vi "camToPipette_abs_3d.vi"(7 "which manipulator":T2(ring), 9 "transform cluster + actuator":T1, 10 "current positions":T3, 11 "abs pixel location":dbl[](array[numeric])) -> (3 "pipette location (steps)":dbl[](array[numeric]))   [LabVIEW 2015]
uses:
  pipette cleaning/pressure box/cleaning_soft/controls/actuator_type.ctl
  pipette cleaning/pressure box/cleaning_soft/controls/actuator_cluster.ctl
  transform_properties_actuators.ctl
  controls/transform_cluster_actuator.ctl
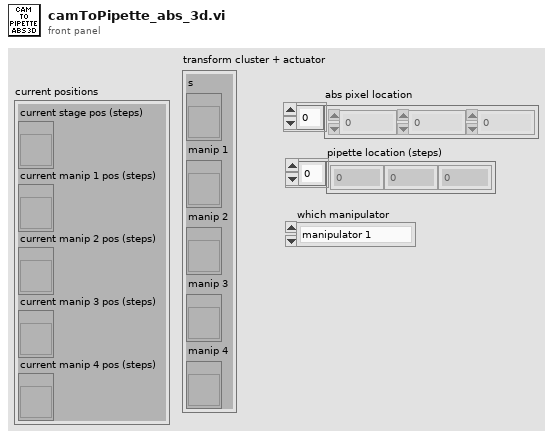
[diagram p1: front panel]
types:
  T1 = typedef "transform_cluster_actuator.ctl" = cluster{"s":refnum<vi>, "manip 1":refnum<vi>, "manip 2":refnum<vi>, "manip 3":refnum<vi>, "manip 4":refnum<vi>}
  T2 = enum16{"manipulator 1", "manipulator 2", "manipulator 3", "manipulator 4"}
  T3 = cluster{"current stage pos (steps)":refnum<vi>, "current manip 1 pos (steps)":refnum<vi>, "current manip 2 pos (steps)":refnum<vi>, "current manip 3 pos (steps)":refnum<vi>, "current manip 4 pos (steps)":refnum<vi>}
  T4 = typedef "transform_properties_actuators.ctl" = cluster{"theta (deg)":dbl, "X sc factor (px/step)":dbl, "Y sc factor (px/step)":dbl, "zero loc (x,y,z)":dbl[], "flip y?":bool, "flip x?":bool, "gamma (deg)":dbl, "flip z?":bool, "Z sc factor (px/step)":dbl, "actuator":T5, "safe space (steps)":i32[]}
  T5 = typedef "actuator_cluster.ctl" = cluster{"Actuator COM":refnum<visa-resource-name>, "Actuator type":T6}
  T6 = typedef "actuator_type.ctl" = enum16{"Scientifica", "Sutter", "Demo", "Off"}
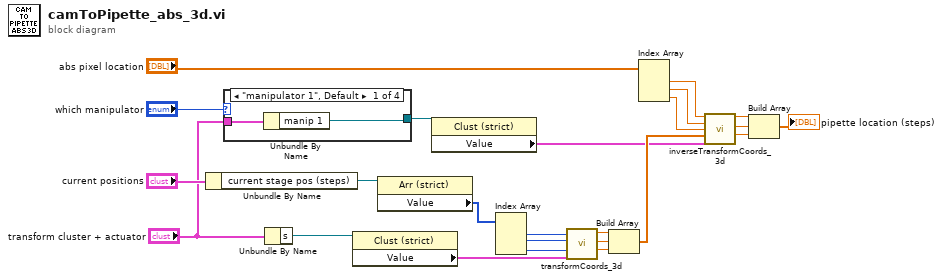
[diagram p0: block diagram]
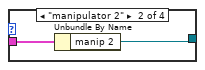
[diagram p2: hidden frame]
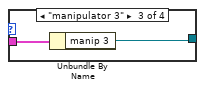
[diagram p3: hidden frame]
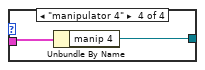
[diagram p4: hidden frame]
diagram:
  n1 = Unbundle By Name("current positions") -> ("current stage pos (steps)"=w20:refnum<vi>)
  n2 = case shown="\"manipulator 1\", Default" "which manipulator" {
    tunnel: "transform cluster + actuator" -> [w26 w28 w30 w32]
    tunnel: [w25 w27 w29 w31] -> w23
    frame "manipulator 1", Default {
      n3 = Unbundle By Name(w26) -> ("manip 1"=w25:refnum<vi>)
    }
    frame "manipulator 2" {
      n4 = Unbundle By Name(w28) -> ("manip 2"=w27:refnum<vi>)
    }
    frame "manipulator 3" {
      n5 = Unbundle By Name(w30) -> ("manip 3"=w29:refnum<vi>)
    }
    frame "manipulator 4" {
      n6 = Unbundle By Name(w32) -> ("manip 4"=w31:refnum<vi>)
    }
  }
  n7 = Unbundle By Name("transform cluster + actuator") -> ("s"=w21:refnum<vi>)
  n8 = property class="Clust (strict)"(reference=w21) -> ("Value"=w18:T4)  [unwired: 1 in, 2 out]
  n9 = property class="Arr (strict)"(reference=w20) -> ("Value"=w19:i32[])  [unwired: 1 in, 2 out]
  n10 = property class="Clust (strict)"(reference=w23) -> ("Value"=w9:T4)  [unwired: 1 in, 2 out]
  n11 = Index Array(array=w19) -> (element #1=w17:i32, element #2=w16:i32, element #3=w4:i32)  [unwired: 3 in]
  n12 = call "transformCoords_3d.vi"("transform properties"=w18, "z"=w4, "y"=w16, "x"=w17) -> ("z out"=w3:dbl, "y out"=w14:dbl, "x out"=w15:dbl)  [unwired: 5 in]
  n13 = Build Array(w15, w14, w3) -> (w10:dbl[])
  n14 = Index Array(array="abs pixel location") -> (element #1=w12:dbl, element #2=w11:dbl, element #3=w2:dbl)  [unwired: 3 in]
  n15 = call "inverseTransformCoords_3d.vi"("x"=w12, "y"=w11, "z"=w2, "current stage pos (px)"=w10, "transform properties"=w9) -> ("x out"=w8:dbl, "y out"=w7:dbl, "z out"=w1:dbl)  [unwired: 8 in]
  n16 = Build Array(w8, w7, w1) -> (→"pipette location (steps)":dbl[])
